vi "getCmdUserEventInstance.vi"(8 "error in (no error)":errorcluster, 11 "tcpServer in":refnum<class "TcpServer.lvclass">) -> (0 "error out":errorcluster, 1 "CmdStatus":refnum<user-event>, 2 "Cmd":refnum<user-event>, 3 "tcpServer out":refnum<class "TcpServer.lvclass">)   [LabVIEW 2018, in "TcpServer.lvclass"]
doc: "Get the command user event instance."
uses:
  TcpServer.lvclass
  typedef/ackTypeDef.ctl
  typedef/tcpPacketTypeDef.ctl
  TcpServer.lvclass/TcpServer.ctl
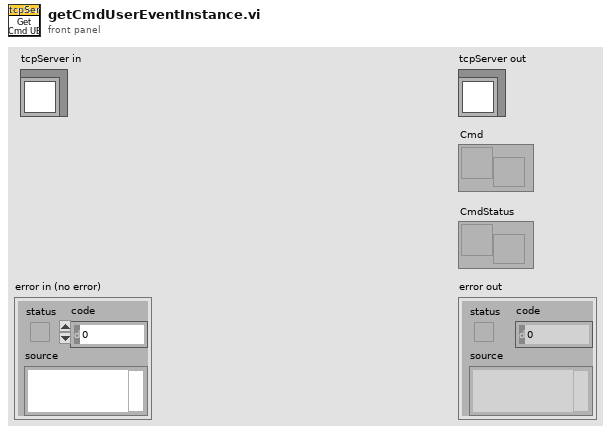
[diagram p1: front panel]
types:
  T1 = typedef "TcpServer.lvclass/userEventsTypeDef.ctl" = cluster{"TcpServer":refnum<user-event>, "Cmd":refnum<user-event>, "CmdStatus":refnum<user-event>, "Event":refnum<user-event>}
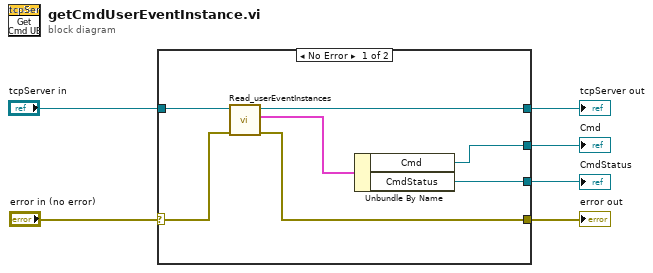
[diagram p0: block diagram]
diagram:
  n1 = case shown="No Error" "error in (no error)" {
    selector: "error in (no error)" -> [w9 w15]
    tunnel: [w8 w15] -> w5
    tunnel: [w12 w14] -> w3
    tunnel: "tcpServer in" -> [w13 w14]
    tunnel: [w10 _] -> w2
    tunnel: [w7 _] -> w1
    frame No Error {
      n2 = call "Read_userEventInstances.vi"("error in (no error)"=w9, "tcpServer in"=w13) -> ("error out"=w8:errorcluster, "UserEvents"=w11:T1, "tcpServer out"=w12:refnum<class "TcpServer.lvclass">)  [unwired: 7 in]
      n3 = Unbundle By Name(w11) -> ("Cmd"=w10:refnum<user-event>, "CmdStatus"=w7:refnum<user-event>)
    }
    frame Error {
    }
  }
  "error out" <- w5
  "tcpServer out" <- w3
  "CmdStatus" <- w1
  "Cmd" <- w2
